vi "EX 9-4 Blink XBOXClick.vi"() -> ()   [LabVIEW 2011]
uses:
  <vilib>/LabVIEW Interface for Arduino/Type Defs/Board Type.ctl
  <vilib>/LabVIEW Interface for Arduino/Type Defs/Connection Type.ctl
  <vilib>/LabVIEW Interface for Arduino/Type Defs/Pin Mode.ctl
  <vilib>/Utility/inputDevices.llb/closeJoystick.vi
  <vilib>/Utility/inputDevices.llb/joystickAcquire.vi
  <vilib>/LabVIEW Interface for Arduino/LabVIEW Interface for Arduino.lvlib
panel:
  out "button info":T1
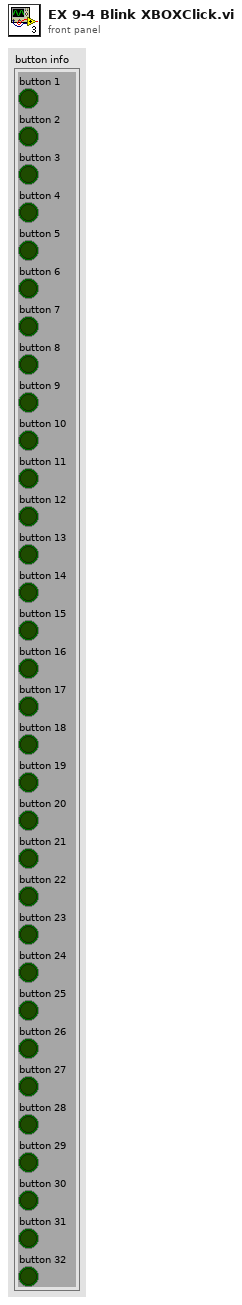
[diagram p1: front panel]
types:
  T1 = cluster{"button 1":bool, "button 2":bool, "button 3":bool, "button 4":bool, "button 5":bool, "button 6":bool, "button 7":bool, "button 8":bool, "button 9":bool, "button 10":bool, "button 11":bool, "button 12":bool, "button 13":bool, "button 14":bool, "button 15":bool, "button 16":bool, "button 17":bool, "button 18":bool, "button 19":bool, "button 20":bool, "button 21":bool, "button 22":bool, "button 23":bool, "button 24":bool, "button 25":bool, "button 26":bool, "button 27":bool, "button 28":bool, "button 29":bool, "button 30":bool, "button 31":bool, "button 32":bool}
  T2 = typedef "LabVIEW Interface for Arduino.lvlib/Pin Mode.ctl" = enum8{"Input", "Output"}
  T3 = typedef "LabVIEW Interface for Arduino.lvlib/Connection Type.ctl" = enum8{"USB / Serial", "XBEE", "BlueSmirf (Bluetooth)"}
  T4 = typedef "LabVIEW Interface for Arduino.lvlib/Board Type.ctl" = enum16{"Uno", "Dimuelanove w/Atmega 328", "Mega 2560"}
  T5 = typedef "LabVIEW Interface for Arduino.lvlib/Arduino Resource.ctl" = cluster{"VISA resource":refnum<visa-resource-name>, "Board Type":T4, "Connection Type":enum8{"USB / Serial"}, "Bytes Per Packet (15)":u8}
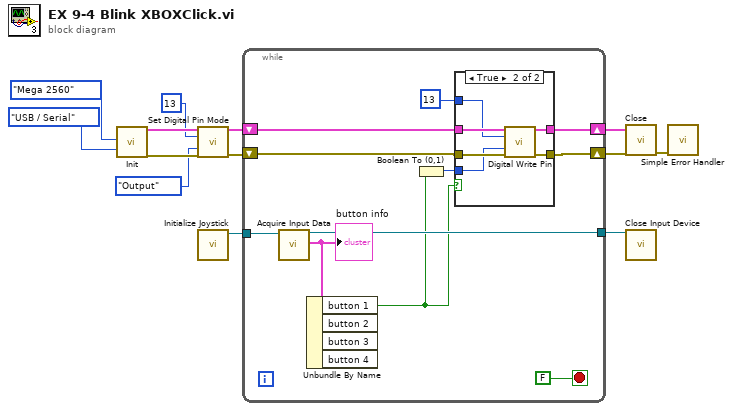
[diagram p0: block diagram]
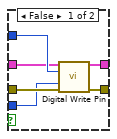
[diagram p2: hidden frame]
diagram:
  n1 = call <vilib>:"Init.vi"("Board Type (Uno)"=Board_Type."Mega 2560", "Connection Type (USB/Serial)"=Connection_Type."USB / Serial") -> ("Arduino Resource"=w6:T5, "error out"=w3:errorcluster)  [unwired: 16 in]
  n2 = call <vilib>:"Set Digital Pin Mode.vi"("Arduino Resource"=w6, "Digital I/O Pin"=u8 13, "Pin Mode (Input)"=Pin_Mode."Output", "error in"=w3) -> ("Arduino Resource"=w5:T5, "error out"=w4:errorcluster)  [unwired: 10 in]
  n3 = call <vilib>:"Initialize Joystick.vi"() -> ("device ID"=w8:refnum<k1>)  [unwired: 10 in, 1 out]
  n4 = while {
    shift-right: [w23] -> w13
    shift-left: w5 -> [w18]
    shift-right: [w22] -> w12
    shift-left: w4 -> [w17]
    tunnel: w8 -> [w21]
    tunnel: [w20] -> w7
    stop <- FALSE stop-if-true
    n5 = call-poly <vilib>:"Acquire Input Data.vi"("device ID"=w21) -> ("device ID"=w20:refnum<k1>, "button info"=w15:T1)  [unwired: 14 in, 3 out]
    "button info" <- w15
    n6 = Unbundle By Name(w15) -> ("button 1"=w14:bool)  [unwired: 3 out]
    n7 = Boolean To (0,1)(Boolean=w14) -> (0, 1=w19:i16)
    n8 = case shown="True" w14 {
      tunnel: w18 -> [w28 w36]
      tunnel: [w27 w35] -> w23
      tunnel: [w26 w34] -> w22
      tunnel: w17 -> [w30 w33]
      tunnel: u8 13 ("Digital I/O Pin") -> [w29 w32]
      tunnel: w19 -> [w25 w31]
      frame False {
        n9 = call <vilib>:"Digital Write Pin.vi"("Arduino Resource"=w28, "Digital I/O Pin (0)"=w29, "Value (0)"=w25, "error in"=w30) -> ("Arduino Resource"=w27:T5, "error out"=w26:errorcluster)  [unwired: 10 in]
      }
      frame True {
        n10 = call <vilib>:"Digital Write Pin.vi"("Arduino Resource"=w36, "Digital I/O Pin (0)"=w32, "Value (0)"=w31, "error in"=w33) -> ("Arduino Resource"=w35:T5, "error out"=w34:errorcluster)  [unwired: 10 in]
      }
    }
  }
  n11 = call <vilib>:"Close.vi"("Arduino Resource"=w13, "error in"=w12) -> ("error out"=w11:errorcluster)  [unwired: 13 in]
  n12 = call-poly <vilib>:"Close Input Device.vi"("device ID"=w7) -> ()  [unwired: 9 in, 1 out]
  n13 = call <vilib>:"Simple Error Handler.vi"("error in (no error)"=w11) -> ()  [unwired: 4 in, 5 out]
